vi "check.vi"() -> ()   [LabVIEW 2010]
panel:
  in  "stop":bool
  in  "Shared Variable Control":refnum<k21>
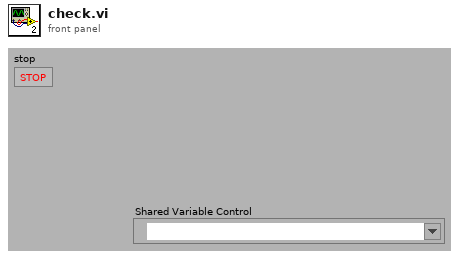
[diagram p1: front panel]
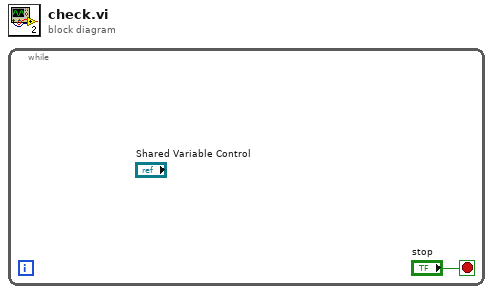
[diagram p0: block diagram]
diagram:
  n1 = while {
    stop <- "stop" stop-if-true
  }
